vi "Control Point Suffix 2 LBCB Number Type.vi"(10 "Contol\nPoint\nSuffix":T2) -> (2 "LBCB Number":T1)   [LabVIEW 2009]
uses:
  Control Point Suffix.ctl
  Data Access Objects/Metadata/LBCB Number.ctl
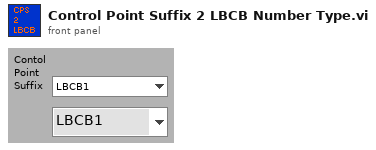
[diagram p1: front panel]
types:
  T1 = typedef "LBCB Number.ctl" = enum16{"LBCB1", "LBCB2"}
  T2 = typedef "Control Point Suffix.ctl" = enum16{"LBCB1", "LBCB2", "ExternalSensors"}
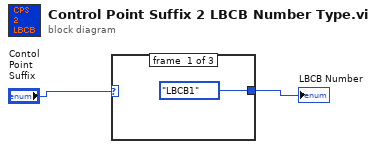
[diagram p0: block diagram]
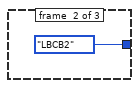
[diagram p2: hidden frame]
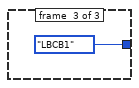
[diagram p3: hidden frame]
diagram:
  n1 = case shown="\"LBCB2\"" "Contol\nPoint\nSuffix" {
    tunnel: [LBCB_Number."LBCB1" ("LBCB Number") LBCB_Number."LBCB2" ("LBCB Number") LBCB_Number."LBCB1" ("LBCB Number")] -> w1
    frame #0 {
    }
    frame #1 {
    }
    frame #2 {
    }
  }
  "LBCB Number" <- w1
